vi "Follow.vi"(8 "error in":errorcluster) -> (0 "error out":errorcluster)   [LabVIEW 2013]
panel:
  out "Joints":dbl[](array[numeric])=[0.0, -45.0, 0.0, 45.0, 0.0, 90.0, 0.0]
  in  "Idle Left":bool
  in  "stop":bool
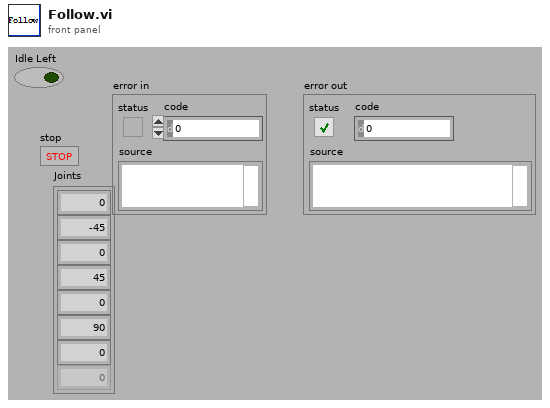
[diagram p1: front panel]
types:
  T1 = typedef "NI_Matrix.lvlib/RealMatrix.ctl" = dbl[][]
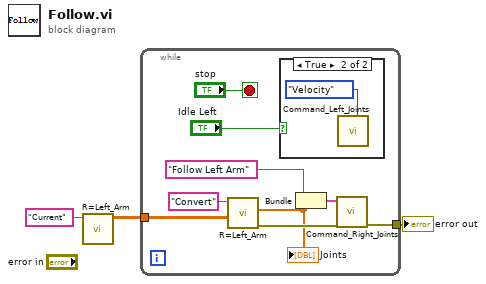
[diagram p0: block diagram]
diagram:
  n1 = call "R=Left_Arm.vi"("Command"="Current") -> ("Matrix"=w2:T1)  [unwired: 8 in, 2 out]
  n2 = while {
    tunnel: w2 -> [w9]
    tunnel: [w4] -> w1
    stop <- "stop" stop-if-true
    n3 = call "R=Left_Arm.vi"("Matrix"=w9, "Command"="Convert") -> ("error out"=w7:errorcluster, "Joints"=w6:dbl[])  [unwired: 7 in, 1 out]
    "Joints" <- w6
    n4 = case shown="True" "Idle Left" {
      frame False {
      }
      frame True {
        n5 = call "Command_Left_Joints.vi"("Mode"=enum32{"Position", "Velocity", "Effort"}."Velocity") -> ()  [unwired: 7 in, 2 out]
      }
    }
    n6 = Bundle("Follow Left Arm", "Joints"=w6) -> (w5:cluster{string, "Joints":dbl[]})  [unwired: 1 in]
    n7 = call "Command_Right_Joints.vi"("error in"=w7, "Goal"=w5) -> ("error out"=w4:errorcluster)  [unwired: 6 in, 1 out]
  }
  "error out" <- w1
